vi "retrieve_motor_state.vi"(0 "device_index (in) [0=def]":i32, 5 "Error In":errorcluster) -> (16 "full_state":T1={"X"={"motion_state"=enum."CONST", "other_states"=[]}, "Y"={"motion_state"=enum."CONST", "other_states"=[]}, "Z"={"motion_state"=enum."CONST", "other_states"=[]}, "U"={"motion_state"=enum."CONST", "other_states"=[]}, "buffer_enabled?"=FALSE, "buffer_start"=0, "buffer_end"=0, "avail_buffer"=0, "move_mode"=enum."ABSOLUTE"}, 19 "Error Out":errorcluster)   [LabVIEW 2013, in "examples.lvlib"]
doc: "Retrieve motor state.\n\nThis VI takes as input an array of polarity \"items\". Each item consists of an item name and an item value. The item name is selectable from list of available polarity definitions that may or may not be applicable to the referenced controller. Please refer to the supporting documenation for the referenced controller if there is any confusion about whether a given polarity item is supported.\n\nProduced By:\n\n<B>Kod Integrations, LLC</B>\n4835 Marianne Drive\nMount Airy, MD 21771\nhttp://www.kodintegrations.com\nemail: info@kodintegrations.com\nphone: (240) 687-1288"
uses:
  libraries/examples.lvlib
  classes/Controller/_Controller.lvclass
  common/controls/axis.ctl
  libraries/common.lvlib
  common/controls/motor_status.ctl
  common/controls/single_axis_state.ctl
  common/controls/move_mode.ctl
  common/controls/complete_motor_state.ctl
panel:
  in  "axis (def=X)":T5
  in  "clear_buffer? (T)":bool=TRUE
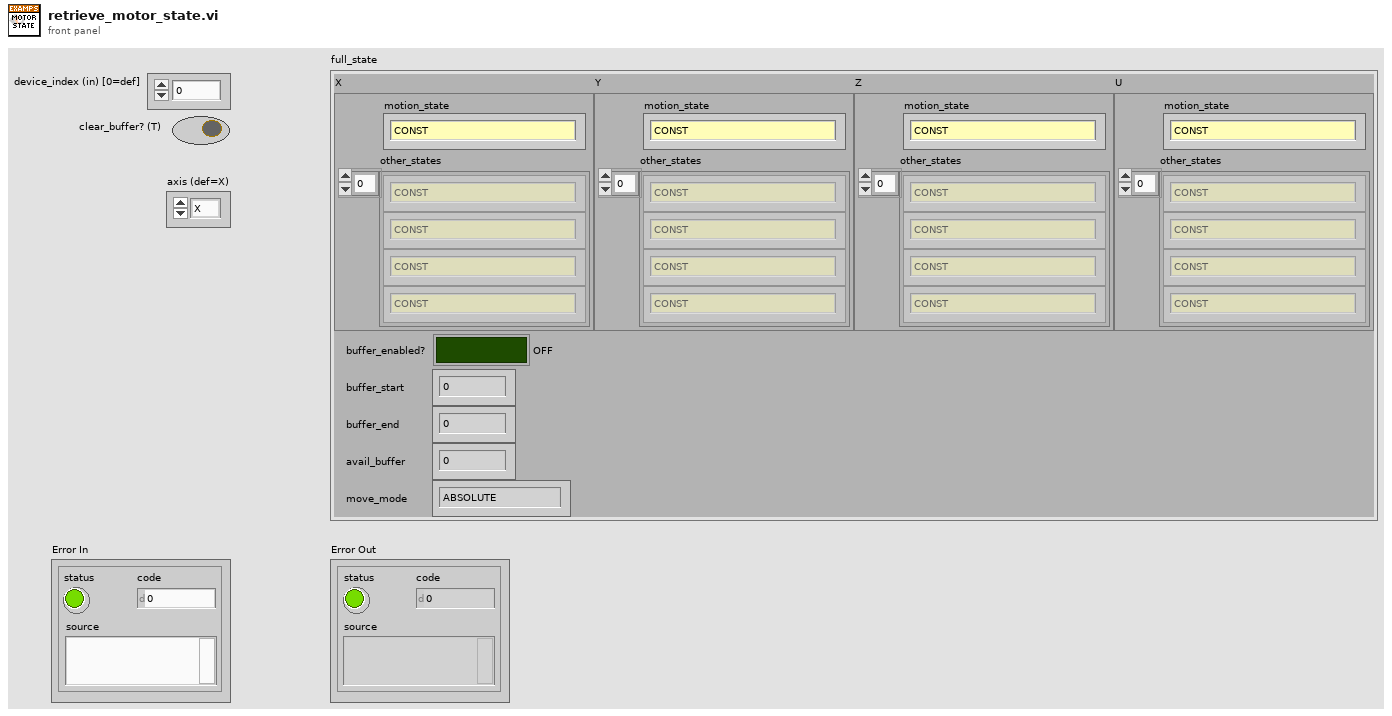
[diagram p1: front panel]
types:
  T1 = typedef "common.lvlib/complete_motor_state.ctl" = cluster{"X":T2, "Y":T2, "Z":T2, "U":T2, "buffer_enabled?":bool, "buffer_start":i32, "buffer_end":i32, "avail_buffer":i32, "move_mode":T4}
  T2 = typedef "common.lvlib/single_axis_state.ctl" = cluster{"motion_state":T3, "other_states":T3[]}
  T3 = typedef "common.lvlib/motor_status.ctl" = enum16{"IDLE", "CONST", "ACCEL", "DECEL", "HOME_SWITCH", "-LIMIT_SWITCH", "+LIMIT_SWITCH", "-LIMIT_ERR", "+LIMIT_ERR", "COMM_TIMEOUT", "ALARM_INPUT", "ALARM_ERROR", "TOC_TIMEOUT_STATUS", "LATCH_INPUT_STATUS", "Z_INDEX_STATUS"}
  T4 = typedef "common.lvlib/move_mode.ctl" = enum16{"ABSOLUTE", "INCREMENTAL"}
  T5 = typedef "common.lvlib/axis.ctl" = enum16{"X", "Y", "Z", "U"}
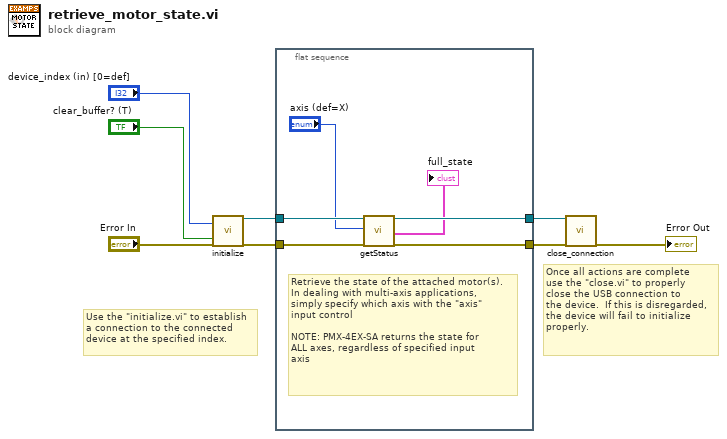
[diagram p0: block diagram]
diagram:
  # "Once all actions are complete\nuse the \"close.vi\" to properly\nclose the USB connection to \nthe device.  If this is disregarded,\nthe device will fail to initialize \nproperly."
  # "Use the \"initialize.vi\" to establish\na connection to the connected\ndevice at the specified index."
  n1 = call "initialize.vi"("device_index (in) [0=def]"="device_index (in) [0=def]", "clear_buffer? (T)"="clear_buffer? (T)", "error in (no error)"="Error In") -> ("reference (out)"=w5:refnum<class "_Controller.lvclass">, "error out"=w4:errorcluster)  [unwired: 15 in]
  n2 = flat-sequence {
    tunnel: w5 -> [w14]
    tunnel: w4 -> [w12]
    tunnel: [w13] -> w3
    tunnel: [w11] -> w2
    frame #0 {
      # "Retrieve the state of the attached motor(s).\nIn dealing with multi-axis applications, \nsimply specify which axis with the \"axis\"\ninput control\n\nNOTE: PMX-4EX-SA returns the state for \nALL axes, regardless of specified input\naxis"
      n3 = call-dynamic "getStatus.vi"("reference (in)"=w14, "axis (def=X)"="axis (def=X)", "error in (no error)"=w12) -> ("reference (out)"=w13:refnum<class "_Controller.lvclass">, "full_state"=→"full_state":T1, "error out"=w11:errorcluster)  [unwired: 13 in, 1 out]
    }
  }
  n4 = call "close_connection.vi"("reference (in)"=w3, "error in (no error)"=w2) -> ("error out"=→"Error Out":errorcluster)  [unwired: 16 in, 1 out]
